vi "ChangeSegment.vi"(8 "error in (no error)":errorcluster, 10 "Message Value":string, 11 "cRef.Configuration.References.ListboxMeasurementArea":refnum<vi>) -> (0 "error out":errorcluster, 2 "Moved?":bool=TRUE, 3 "target out":path)   [LabVIEW 2013, in "main.lvlib"]
uses:
  main.lvlib
  <vilib>/regexp/Match Regular Expression.xnode
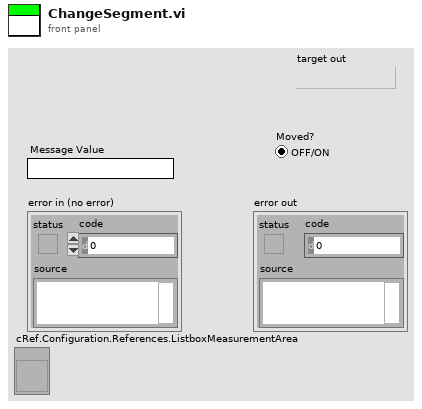
[diagram p1: front panel]
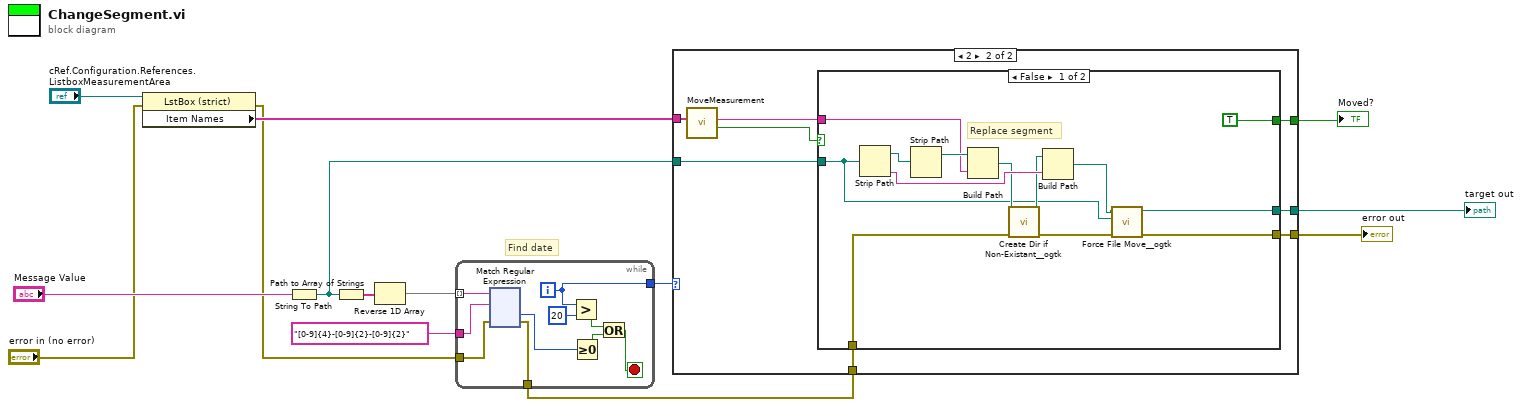
[diagram p0: block diagram]
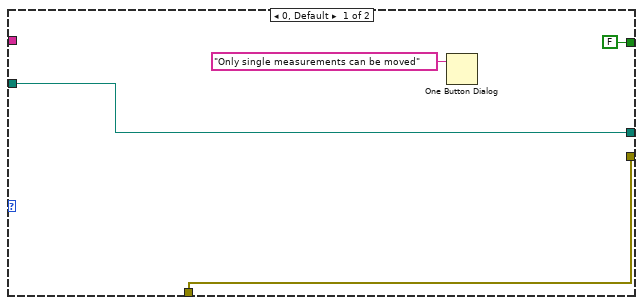
[diagram p2: hidden frame]
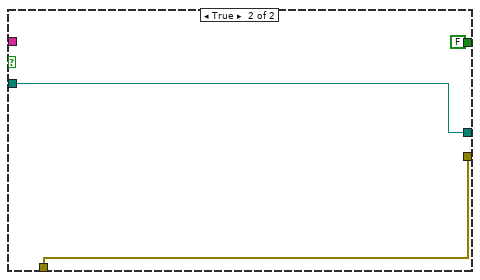
[diagram p3: hidden frame]
diagram:
  # "Find date"
  n1 = property class="LstBox (strict)"(reference="cRef.Configuration.References.ListboxMeasurementArea", error in="error in (no error)") -> (error out=w1:errorcluster, "Item Names"=w3:string[])  [unwired: 1 out]
  n2 = String To Path(string="Message Value") -> (path=w11:path)
  n3 = Path to Array of Strings(0:w11) -> (2:w7:string[])  [unwired: 1 out]
  n4 = Reverse 1D Array(array=w7) -> (reversed array=w8:string[])
  n5 = while {
    tunnel: [w24] -> w10
    tunnel: w8 -> [w20] mode=indexing
    tunnel: w1 -> [w19]
    tunnel: [w17] -> w12
    tunnel: "[0-9]{4}-[0-9]{2}-[0-9]{2}" ("regular expression") -> [w16]
    i -> [w24]
    stop <- w15 stop-if-true
    n6 = xnode "Match Regular Expression"("input string"=w20, "regular expression"=w16, "error in"=w19) -> ("offset past match"=w18:i32, "error out"=w17:errorcluster)  [unwired: 3 in, 3 out]
    n7 = Greater?(x=w24, y=20) -> (0:w21:bool)
    n8 = Greater Or Equal To 0?(x=w18) -> (x >= 0?=w22:bool)
    n9 = Or(x=w21, y=w22) -> (x .or. y?=w15:bool)
  }
  n10 = case shown="2" w10 {
    tunnel: w3 -> [_ w147]
    tunnel: w11 -> [w137 w144]
    tunnel: w12 -> [w138 w143]
    tunnel: [w138 w142] -> w13
    tunnel: [w137 w141] -> w6
    tunnel: [FALSE w140] -> w5
    frame 0, Default {
      n11 = One Button Dialog(message="Only single measurements can be moved") -> ()  [unwired: 1 in, 1 out]
    }
    frame 2 {
      n12 = call "MoveMeasurement.vi"("Strings []"=w147) -> ("Cancel?"=w146:bool, "Segment Out"=w145:string)  [unwired: 9 in]
      n13 = case shown="False" w146 {
        tunnel: w145 -> [w158 _]
        tunnel: w144 -> [w152 w162]
        tunnel: w143 -> [w156 w163]
        tunnel: [w150 w163] -> w142
        tunnel: [w149 w162] -> w141
        tunnel: [TRUE FALSE] -> w140
        frame False {
          # "Replace segment"
          n14 = Strip Path(path=w152) -> (stripped path=w160:path, name=w157:string)
          n15 = Strip Path(path=w160) -> (stripped path=w159:path)  [unwired: 1 out]
          n16 = Build Path(base path=w159, name or relative path=w158) -> (appended path=w155:path)
          n17 = call <userlib>:"Create Dir if Non-Existant__ogtk.vi"("error in (no error)"=w156, "Directory Path"=w155) -> ("error out"=w151:errorcluster, "dup Directory Path"=w154:path)  [unwired: 7 in, 1 out]
          n18 = Build Path(base path=w154, name or relative path=w157) -> (appended path=w153:path)
          n19 = call <userlib>:"Force File Move__ogtk.vi"("error in (no error)"=w151, "source"=w152, "target"=w153) -> ("error out"=w150:errorcluster, "target out"=w149:path)  [unwired: 3 in]
        }
        frame True {
        }
      }
    }
  }
  "error out" <- w13
  "Moved?" <- w5
  "target out" <- w6
